vi "Read ItemObjs.vi"(11 "BetterHandle in":refnum<class "BetterHandle.lvclass">) -> (2 "ItemObjs":refnum<class "BetterItem.lvclass">[](array[class]), 3 "BetterHandle out":refnum<class "BetterHandle.lvclass">)   [LabVIEW 2020, in "BetterDragAndDrop.lvlib" / "BetterHandle.lvclass"]
uses:
  BetterHandle.lvclass
  BetterTreeItem/BetterItem.lvclass
  BetterHandle.lvclass/BetterHandle.ctl
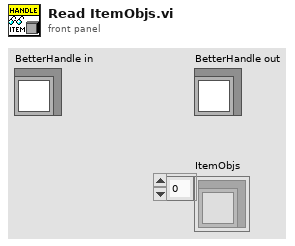
[diagram p1: front panel]
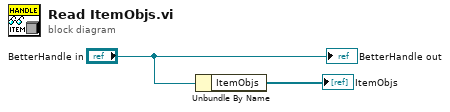
[diagram p0: block diagram]
diagram:
  n1 = Unbundle By Name("BetterHandle in") -> ("ItemObjs"=→"ItemObjs":refnum<class "BetterItem.lvclass">[])
  "BetterHandle out" <- "BetterHandle in"
